vi "determineClassPrivateDataDefaultValue.vi"(8 "error in (no error)":errorcluster, 10 "className":string) -> (0 "error out":errorcluster, 1 "privateDataClusterLabel":string, 2 "privateDataDefaultValue":variant)   [LabVIEW 2020, in "openg_variant.lvlib" / "Reflection.lvclass"]
doc: "Given a classname, output the classes private data default value as a variant cluster.\n\nGCraftsman JSON Object Serialization Toolkit\nwww.GCraftsman.com\nCopyright (c) 2017, GCraftsman"
uses:
  Reflection.lvclass
  Reflection.lvclass/Reflection.ctl
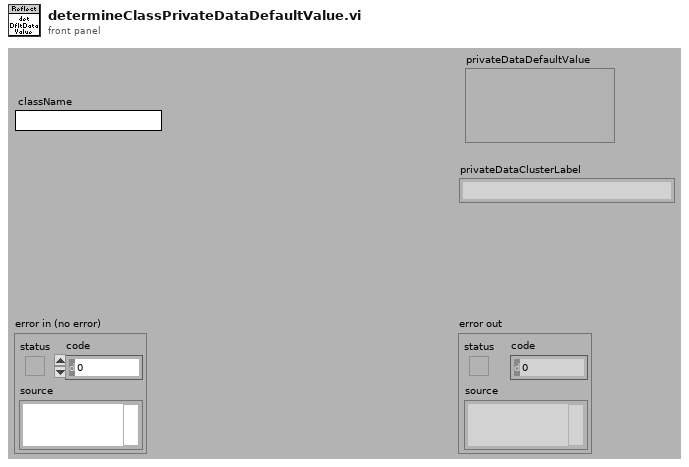
[diagram p1: front panel]
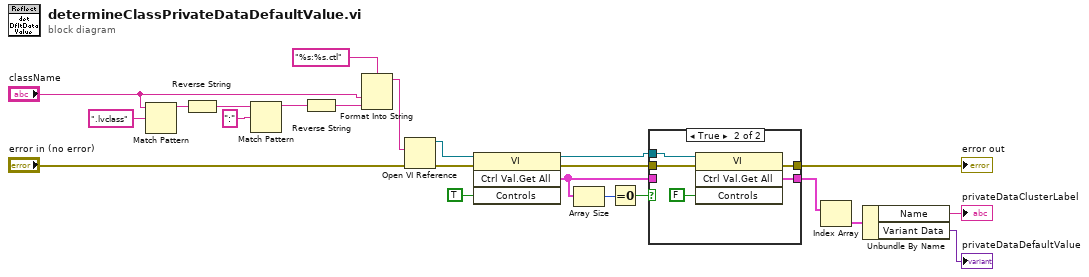
[diagram p0: block diagram]
diagram:
  n1 = Match Pattern(string="className", regular expression=".lvclass") -> (before substring=w5:string)  [unwired: 1 in, 3 out]
  n2 = Reverse String(1:w5) -> (0:w4:string)
  n3 = Match Pattern(string=w4, regular expression=":") -> (before substring=w3:string)  [unwired: 1 in, 3 out]
  n4 = Reverse String(1:w3) -> (0:w2:string)
  n5 = Format Into String(format string="%s:%s.ctl", "className", w2) -> (resulting string=w22:string)  [unwired: 2 in, 1 out]
  n6 = Open VI Reference(vi path=w22, error in (no error)="error in (no error)") -> (vi reference=w21:refnum<vi>, error out=w17:errorcluster)  [unwired: 4 in]
  n7 = invoke class="VI" method="Ctrl Val.Get All"(reference=w21, error in=w17, "Controls"=TRUE) -> (reference out=w14:refnum<vi>, error out=w15:errorcluster, "Get All Control Values Variant"=w10:cluster{"Name":string, "Variant Data":variant}[])  [unwired: 1 in, 1 out]
  n8 = Array Size(array=w10) -> (size(s)=w12:i32)
  n9 = Equal To 0?(x=w12) -> (x = 0?=w11:bool)
  n10 = case shown="True" w11 {
    tunnel: w15 -> [w24 w30]
    tunnel: w14 -> [_ w29]
    tunnel: [w24 w28] -> w13
    tunnel: w10 -> [w25 _]
    tunnel: [w25 w27] -> w9
    frame False {
    }
    frame True {
      n11 = invoke class="VI" method="Ctrl Val.Get All"(reference=w29, error in=w30, "Controls"=FALSE) -> (error out=w28:errorcluster, "Get All Control Values Variant"=w27:cluster{"Name":string, "Variant Data":variant}[])  [unwired: 1 in, 2 out]
    }
  }
  "error out" <- w13
  n12 = Index Array(array=w9) -> (element=w20:cluster{"Name":string, "Variant Data":variant})  [unwired: 1 in]
  n13 = Unbundle By Name(w20) -> ("Name"=→"privateDataClusterLabel":string, "Variant Data"=→"privateDataDefaultValue":variant)
